vi "Error Converter (ErrCode or Status).vi"(0 "error code":i32, 5 "VID":u32=1240 format="%.0x", 7 "PID":u32=221 format="%.0x", 9 "Serial No (max 10 Char)":string, 11 "error in (no error)":errorcluster, 12 "index":i32) -> (15 "error out":errorcluster)   [LabVIEW 2020]
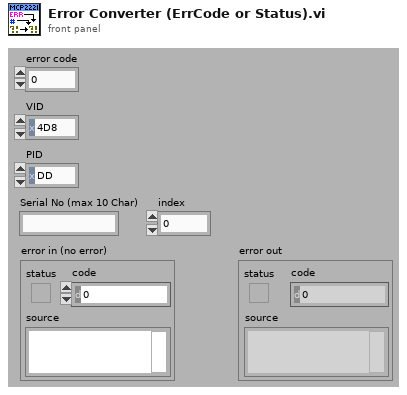
[diagram p1: front panel]
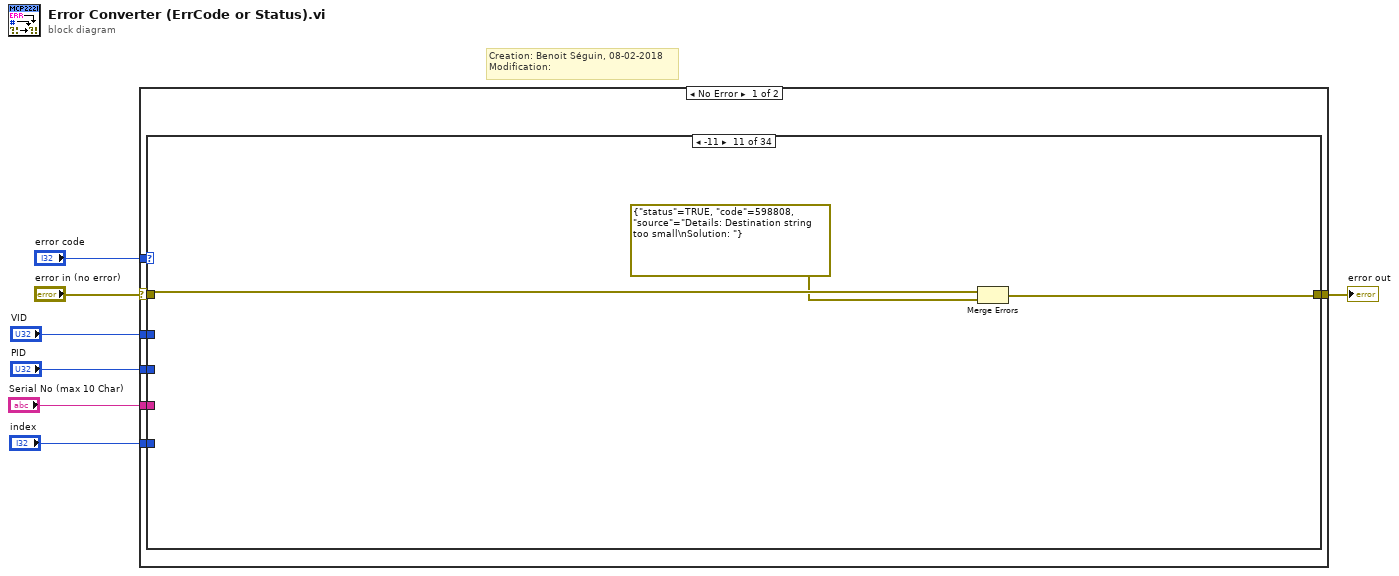
[diagram p0: block diagram]
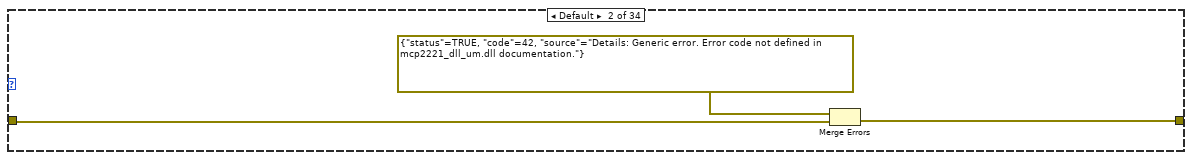
[diagram p3: hidden frame]
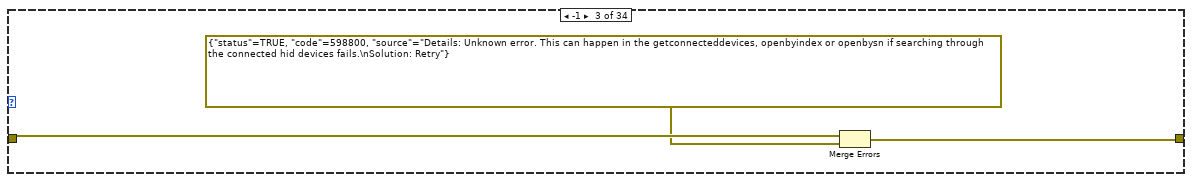
[diagram p4: hidden frame]
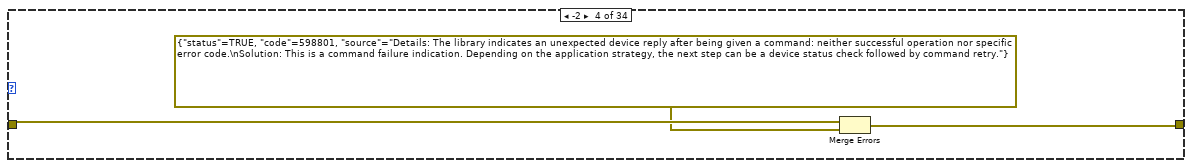
[diagram p5: hidden frame]
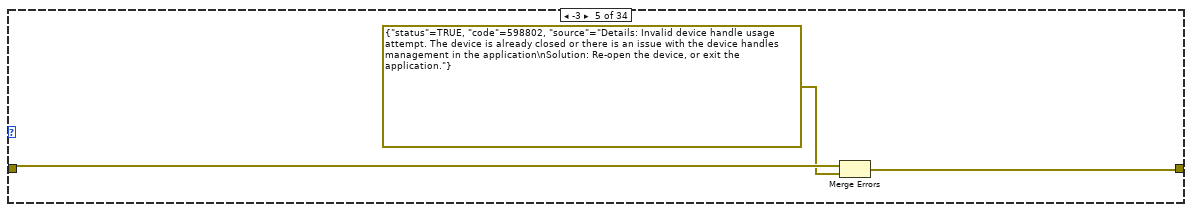
[diagram p6: hidden frame]
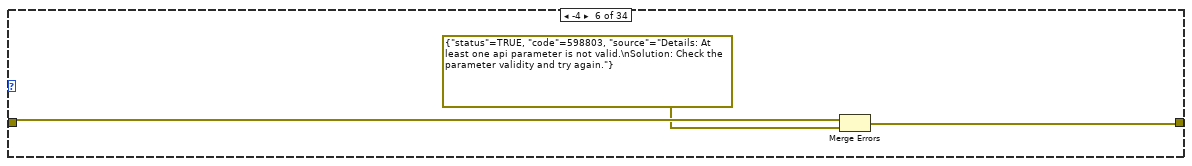
[diagram p7: hidden frame]
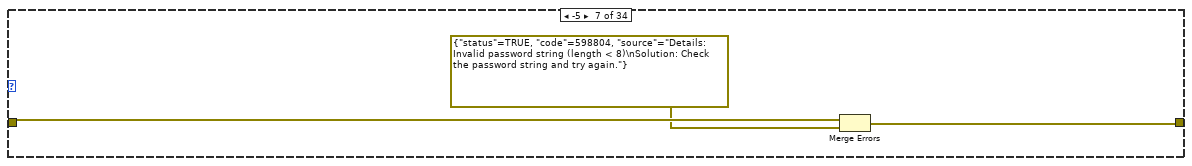
[diagram p8: hidden frame]
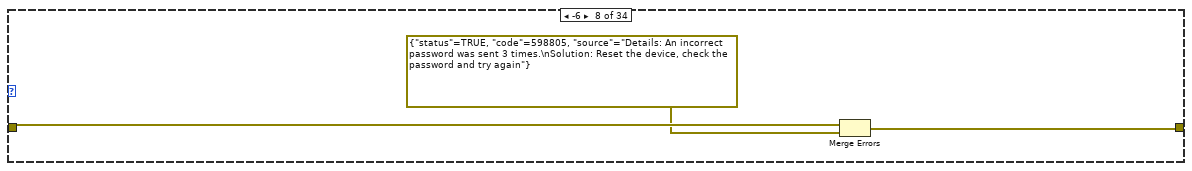
[diagram p9: hidden frame]
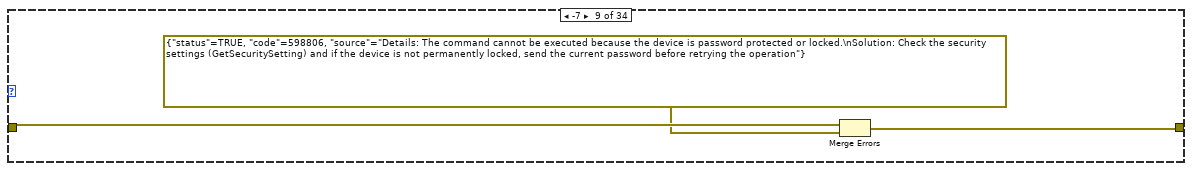
[diagram p10: hidden frame]
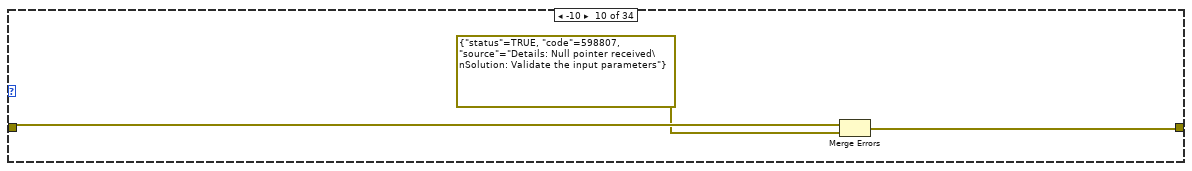
[diagram p11: hidden frame]
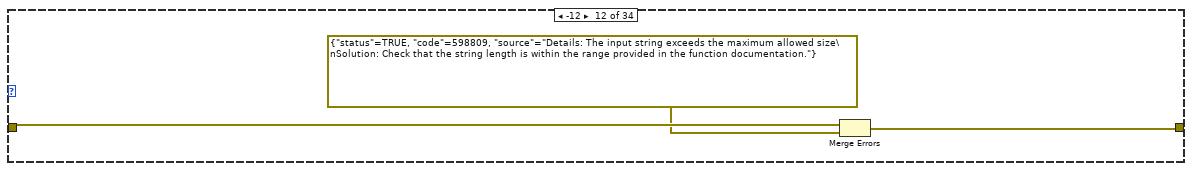
[diagram p12: hidden frame]
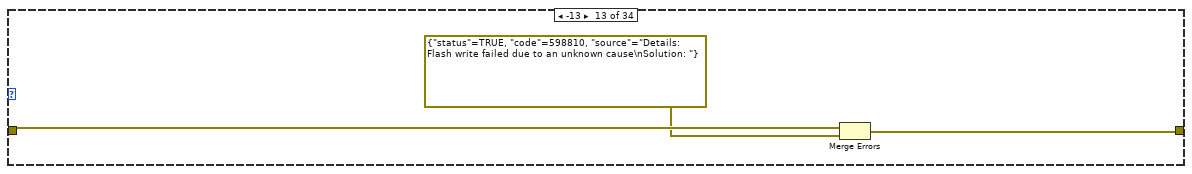
[diagram p13: hidden frame]
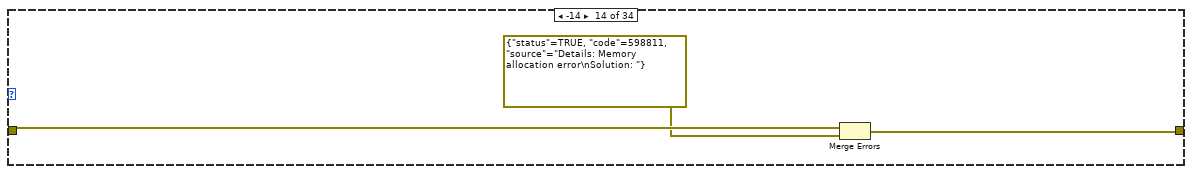
[diagram p14: hidden frame]
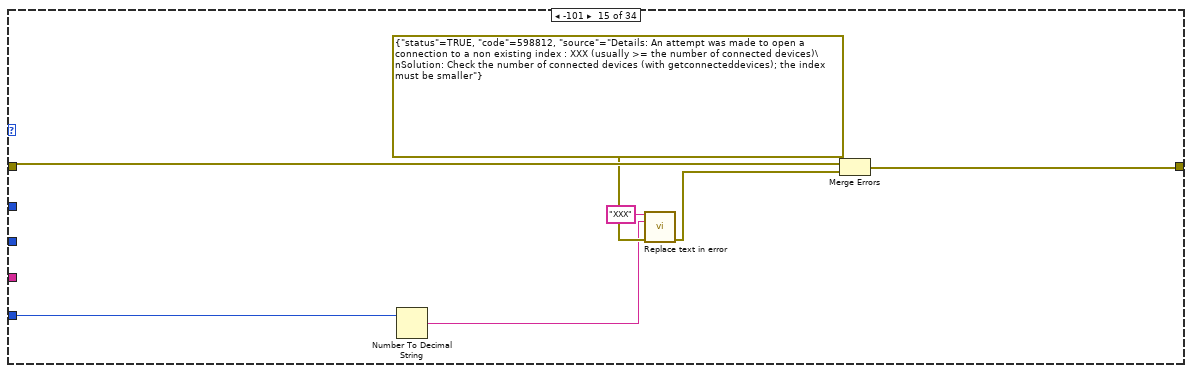
[diagram p15: hidden frame]
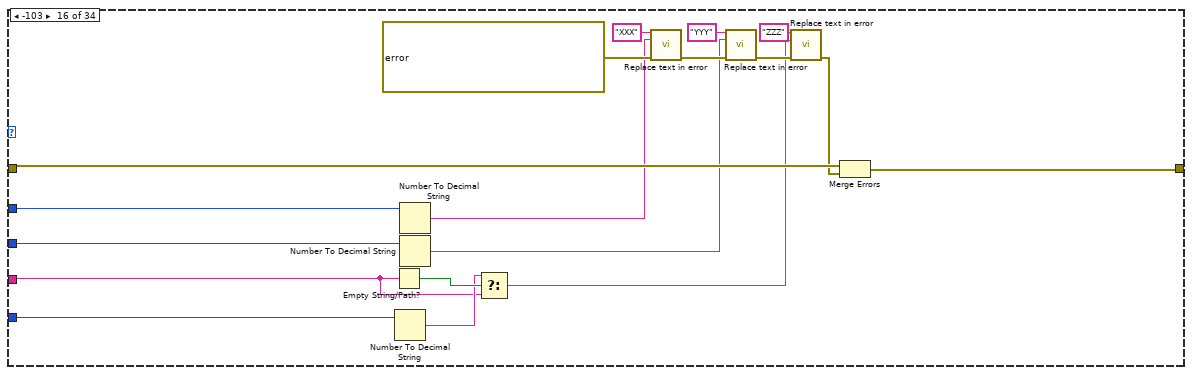
[diagram p16: hidden frame]
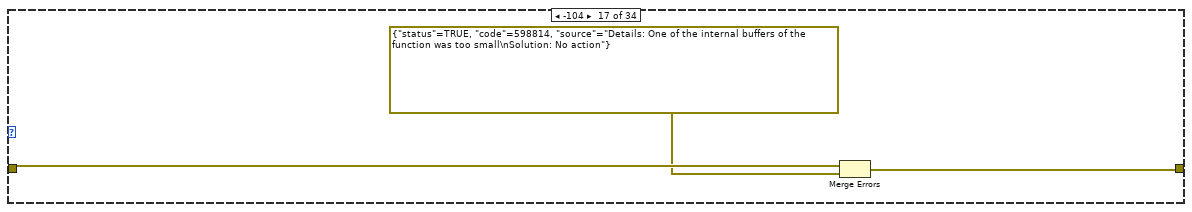
[diagram p17: hidden frame]
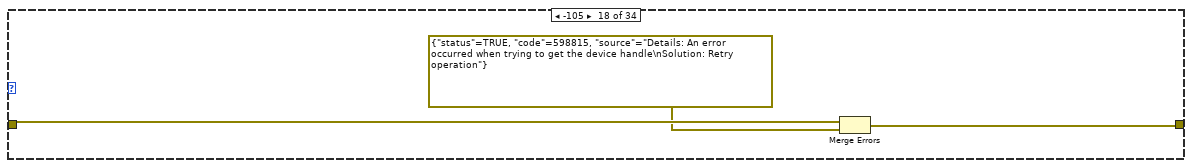
[diagram p18: hidden frame]
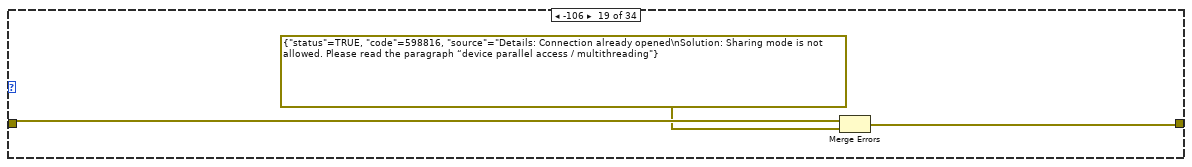
[diagram p19: hidden frame]
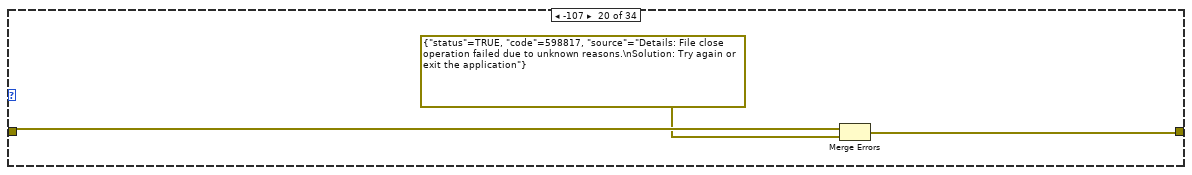
[diagram p20: hidden frame]
diagram:
  # "Creation: Benoit Séguin, 08-02-2018\nModification:"
  n1 = case shown="No Error" "error in (no error)" {
    selector: "error in (no error)" -> [w14 w134]
    tunnel: [w13 w134] -> w5
    tunnel: "error code" -> [w12 _]
    tunnel: "VID" -> [w11 _]
    tunnel: "PID" -> [w10 _]
    tunnel: "Serial No (max 10 Char)" -> [w9 _]
    tunnel: "index" -> [w8 _]
    frame No Error {
      n2 = case shown="-11" w12 {
        tunnel: w14 -> [w15 w17 w20 w23 w26 w29 w32 w35 w38 w41 w44 w47 w50 w53 w60 w78 w81 w84 w87 w90 w93 w96 w99 w102 w105 w108 w111 w114 w117 w120 w123 w126 w129 w132]
        tunnel: [w15 w18 w21 w24 w27 w30 w33 w36 w39 w42 w45 w48 w51 w54 w61 w79 w82 w85 w88 w91 w94 w97 w100 w103 w106 w109 w112 w115 w118 w121 w124 w127 w130 w133] -> w13
        tunnel: w11 -> [_ _ _ _ _ _ _ _ _ _ _ _ _ _ _ w71 _ _ _ _ _ _ _ _ _ _ _ _ _ _ _ _ _ _]
        tunnel: w10 -> [_ _ _ _ _ _ _ _ _ _ _ _ _ _ _ w70 _ _ _ _ _ _ _ _ _ _ _ _ _ _ _ _ _ _]
        tunnel: w9 -> [_ _ _ _ _ _ _ _ _ _ _ _ _ _ _ w64 _ _ _ _ _ _ _ _ _ _ _ _ _ _ _ _ _ _]
        tunnel: w8 -> [_ _ _ _ _ _ _ _ _ _ _ _ _ _ w56 w67 _ _ _ _ _ _ _ _ _ _ _ _ _ _ _ _ _ _]
        frame 0 {
        }
        frame Default {
          n3 = Merge Errors(errorcluster {"status"=TRUE, "code"=42, "source"="Details: Generic error. Error code not defined in mcp2221_dll_um.dll documentation."} ("error in"), w17) -> (w18:errorcluster)
        }
        frame -1 {
          n4 = Merge Errors(w20, errorcluster {"status"=TRUE, "code"=598800, "source"="Details: Unknown error. This can happen in the getconnecteddevices, openbyindex or openbysn if searching through the connected hid devices fails.\nSolution: Retry"} ("error IO")) -> (w21:errorcluster)
        }
        frame -2 {
          n5 = Merge Errors(w23, errorcluster {"status"=TRUE, "code"=598801, "source"="Details: The library indicates an unexpected device reply after being given a command: neither successful operation nor specific error code.\nSolution: This is a command failure indication. Depending on the application strategy, the next step can be a device status check followed by command retry."} ("error IO")) -> (w24:errorcluster)
        }
        frame -3 {
          n6 = Merge Errors(w26, errorcluster {"status"=TRUE, "code"=598802, "source"="Details: Invalid device handle usage attempt. The device is already closed or there is an issue with the device handles management in the application\nSolution: Re-open the device, or exit the application."} ("error IO")) -> (w27:errorcluster)
        }
        frame -4 {
          n7 = Merge Errors(w29, errorcluster {"status"=TRUE, "code"=598803, "source"="Details: At least one api parameter is not valid.\nSolution: Check the parameter validity and try again."} ("error IO")) -> (w30:errorcluster)
        }
        frame -5 {
          n8 = Merge Errors(w32, errorcluster {"status"=TRUE, "code"=598804, "source"="Details: Invalid password string (length < 8)\nSolution: Check the password string and try again."} ("error IO")) -> (w33:errorcluster)
        }
        frame -6 {
          n9 = Merge Errors(w35, errorcluster {"status"=TRUE, "code"=598805, "source"="Details: An incorrect password was sent 3 times.\nSolution: Reset the device, check the password and try again"} ("error IO")) -> (w36:errorcluster)
        }
        frame -7 {
          n10 = Merge Errors(w38, errorcluster {"status"=TRUE, "code"=598806, "source"="Details: The command cannot be executed because the device is password protected or locked.\nSolution: Check the security settings (GetSecuritySetting) and if the device is not permanently locked, send the current password before retrying the operation"} ("error IO")) -> (w39:errorcluster)
        }
        frame -10 {
          n11 = Merge Errors(w41, errorcluster {"status"=TRUE, "code"=598807, "source"="Details: Null pointer received\nSolution: Validate the input parameters"} ("error IO")) -> (w42:errorcluster)
        }
        frame -11 {
          n12 = Merge Errors(w44, errorcluster {"status"=TRUE, "code"=598808, "source"="Details: Destination string too small\nSolution: "} ("error IO")) -> (w45:errorcluster)
        }
        frame -12 {
          n13 = Merge Errors(w47, errorcluster {"status"=TRUE, "code"=598809, "source"="Details: The input string exceeds the maximum allowed size\nSolution: Check that the string length is within the range provided in the function documentation."} ("error IO")) -> (w48:errorcluster)
        }
        frame -13 {
          n14 = Merge Errors(w50, errorcluster {"status"=TRUE, "code"=598810, "source"="Details: Flash write failed due to an unknown cause\nSolution: "} ("error IO")) -> (w51:errorcluster)
        }
        frame -14 {
          n15 = Merge Errors(w53, errorcluster {"status"=TRUE, "code"=598811, "source"="Details: Memory allocation error\nSolution: "} ("error IO")) -> (w54:errorcluster)
        }
        frame -101 {
          n16 = Number To Decimal String(number=w56) -> (decimal integer string=w55:string)  [unwired: 1 in]
          n17 = call "Replace text in error.vi"("Text to find"="XXX", "Replace with"=w55, "error in (no error)"=errorcluster {"status"=TRUE, "code"=598812, "source"="Details: An attempt was made to open a connection to a non existing index : XXX (usually >= the number of connected devices)\nSolution: Check the number of connected devices (with getconnecteddevices); the index must be smaller"} ("error IO")) -> ("error out"=w58:errorcluster)  [unwired: 12 in]
          n18 = Merge Errors(w60, w58) -> (w61:errorcluster)
        }
        frame -103 {
          n19 = Empty String/Path?(string/path=w64) -> (empty?=w66:bool)
          n20 = Number To Decimal String(number=w67) -> (decimal integer string=w65:string)  [unwired: 1 in]
          n21 = Number To Decimal String(number=w71) -> (decimal integer string=w69:string)  [unwired: 1 in]
          n22 = Number To Decimal String(number=w70) -> (decimal integer string=w68:string)  [unwired: 1 in]
          n23 = Select(t=w65, s=w66, f=w64) -> (s? t:f=w63:string)
          n24 = call "Replace text in error.vi"("Text to find"="XXX", "Replace with"=w69, "error in (no error)"=errorcluster {"status"=TRUE, "code"=598813, "source"="Details: No device with the provided vid: XXX or pid: YYY or SN: ZZZ has been found. This error can also occur during i2c/smbus operations if the device is disconnected from the usb before the operation is complete. The OpenBySn method will also return this code if a connection to a matching device is already open.\nSolution:  If Serial number is used set Mcp2221 Set Serial Number Enumeration Enable at TRUE and disconnect and reconnect the device."} ("error IO")) -> ("error out"=w75:errorcluster)  [unwired: 12 in]
          n25 = call "Replace text in error.vi"("Text to find"="YYY", "Replace with"=w68, "error in (no error)"=w75) -> ("error out"=w73:errorcluster)  [unwired: 12 in]
          n26 = call "Replace text in error.vi"("Text to find"="ZZZ", "Replace with"=w63, "error in (no error)"=w73) -> ("error out"=w62:errorcluster)  [unwired: 12 in]
          n27 = Merge Errors(w78, w62) -> (w79:errorcluster)
        }
        frame -104 {
          n28 = Merge Errors(w81, errorcluster {"status"=TRUE, "code"=598814, "source"="Details: One of the internal buffers of the function was too small\nSolution: No action"} ("error IO")) -> (w82:errorcluster)
        }
        frame -105 {
          n29 = Merge Errors(w84, errorcluster {"status"=TRUE, "code"=598815, "source"="Details: An error occurred when trying to get the device handle\nSolution: Retry operation"} ("error IO")) -> (w85:errorcluster)
        }
        frame -106 {
          n30 = Merge Errors(w87, errorcluster {"status"=TRUE, "code"=598816, "source"="Details: Connection already opened\nSolution: Sharing mode is not allowed. Please read the paragraph “device parallel access / multithreading"} ("error IO")) -> (w88:errorcluster)
        }
        frame -107 {
          n31 = Merge Errors(w90, errorcluster {"status"=TRUE, "code"=598817, "source"="Details: File close operation failed due to unknown reasons.\nSolution: Try again or exit the application"} ("error IO")) -> (w91:errorcluster)
        }
        frame -301 {
          n32 = Merge Errors(w93, errorcluster {"status"=TRUE, "code"=598818, "source"="Details: Low level communication error, shouldn't appear during normal operation\nSolution: Restart application"} ("error IO")) -> (w94:errorcluster)
        }
        frame -302 {
          n33 = Merge Errors(w96, errorcluster {"status"=TRUE, "code"=598819, "source"="Details: Low level communication error, shouldn't appear during normal operation\nSolution: Restart application"} ("error IO")) -> (w97:errorcluster)
        }
        frame -303 {
          n34 = Merge Errors(w99, errorcluster {"status"=TRUE, "code"=598820, "source"="Details: Low level communication error shouldn't appear during normal\nSolution: Restart application"} ("error IO")) -> (w100:errorcluster)
        }
        frame -401 {
          n35 = Merge Errors(w102, errorcluster {"status"=TRUE, "code"=598821, "source"="Details: I2c/smbus speed is not within accepted range of 46875 - 500000\nSolution: "} ("error IO")) -> (w103:errorcluster)
        }
        frame -402 {
          n36 = Merge Errors(w105, errorcluster {"status"=TRUE, "code"=598822, "source"="Details: The speed may fail to be set if an i2c/smbus operation is already in progress or in a timeout situation. The \"mcp2221_i2ccancelcurrenttransfer\" function can be used to free the bus before retrying to set the speed.\nSolution: "} ("error IO")) -> (w106:errorcluster)
        }
        frame -403 {
          n37 = Merge Errors(w108, errorcluster {"status"=TRUE, "code"=598823, "source"="Details: The byte count is outside the accepted range for the attempted operation\nSolution: Check the valid range for the desired operation and retry"} ("error IO")) -> (w109:errorcluster)
        }
        frame -404 {
          n38 = Merge Errors(w111, errorcluster {"status"=TRUE, "code"=598824, "source"="Details: Invalid slave address. If 7 bit addressing is used the maximum address value is 127\nSolution: "} ("error IO")) -> (w112:errorcluster)
        }
        frame -405 {
          n39 = Merge Errors(w114, errorcluster {"status"=TRUE, "code"=598825, "source"="Details: The mcp2221 i2c/smbus engine is currently busy.\nSolution: Retry operation or call cancelcurrenti2ctransfer before another retry."} ("error IO")) -> (w115:errorcluster)
        }
        frame -406 {
          n40 = Merge Errors(w117, errorcluster {"status"=TRUE, "code"=598826, "source"="Details: Mcp2221 signaled an error during the i2c read operation\nSolution: Retry or reset device before retrying"} ("error IO")) -> (w118:errorcluster)
        }
        frame -407 {
          n41 = Merge Errors(w120, errorcluster {"status"=TRUE, "code"=598827, "source"="Details: Nack received for the slave address used\nSolution: Check that the slave address is correct."} ("error IO")) -> (w121:errorcluster)
        }
        frame -408 {
          n42 = Merge Errors(w123, errorcluster {"status"=TRUE, "code"=598828, "source"="Details: Either the \"timeout\" or \"retries\" value has been exceeded and no reply was received from the slave.\nSolution: I2c/smbus transfer is not working properly. Check the communication settings and try again. The retries and timeout values can also be updated in the SetAdvancedCommParams"} ("error IO")) -> (w124:errorcluster)
        }
        frame -409 {
          n43 = Merge Errors(w126, errorcluster {"status"=TRUE, "code"=598829, "source"="Details: The number of received data bytes is greater than requested\nSolution: "} ("error IO")) -> (w127:errorcluster)
        }
        frame -410 {
          n44 = Merge Errors(w129, errorcluster {"status"=TRUE, "code"=598830, "source"="Details: Could not copy the data received from the slave into the provided buffer;\nSolution: Check buffer size and retry operation"} ("error IO")) -> (w130:errorcluster)
        }
        frame -411 {
          n45 = Merge Errors(w132, errorcluster {"status"=TRUE, "code"=598831, "source"="Details: The i2c engine (inside mcp2221) was already idle. The cancellation command had no effect.\nSolution: "} ("error IO")) -> (w133:errorcluster)
        }
      }
    }
    frame Error {
    }
  }
  "error out" <- w5
